vi "loadMapping.vi"(8 "error in (no error)":errorcluster, 9 "xmlPath":string, 10 "channel_configXML":refnum<class "NativeXML.lvclass">, 11 "Channel in":refnum<class "Channel.lvclass">) -> (0 "error out":errorcluster, 3 "Channel out":refnum<class "Channel.lvclass">)   [LabVIEW 2011, in "Tools.lvlib" / "DatabaseHelpers.lvlib" / "Channel.lvclass"]
uses:
  Channel.lvclass
  NativeXML/NativeXML.lvclass
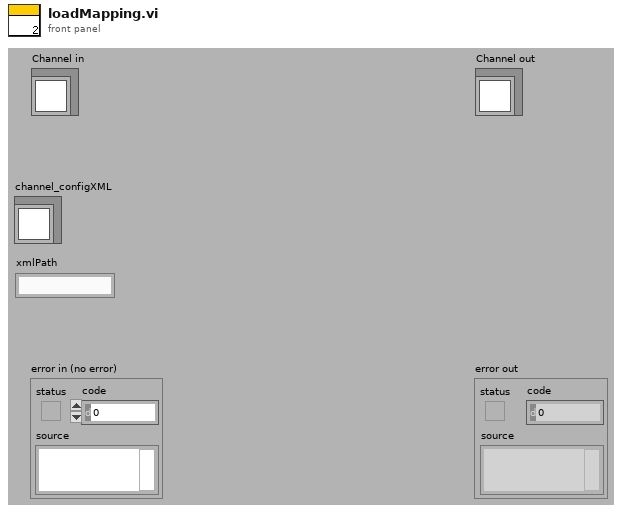
[diagram p1: front panel]
types:
  T1 = cluster{"Attribute String":string, "Value":string}
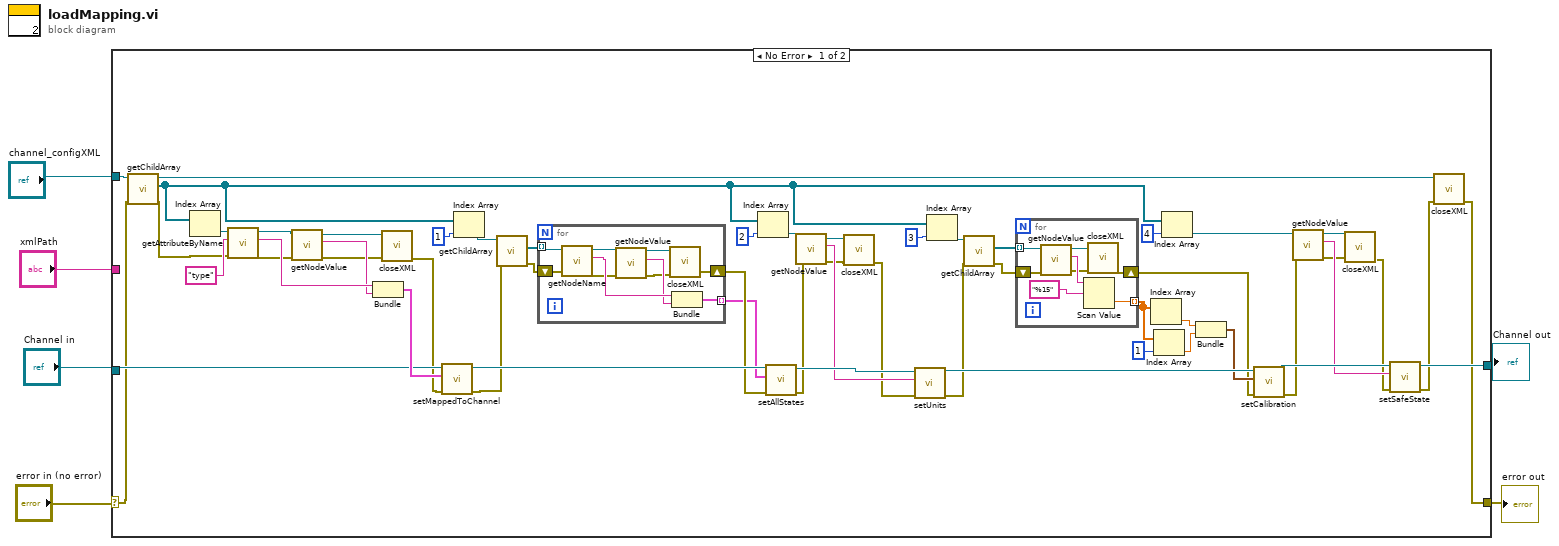
[diagram p0: block diagram]
diagram:
  n1 = case shown="No Error" "error in (no error)" {
    selector: "error in (no error)" -> [w41 w81]
    tunnel: [w7 w81] -> w4
    tunnel: "channel_configXML" -> [w43 _]
    tunnel: "Channel in" -> [w60 w80]
    tunnel: [w44 w80] -> w3
    tunnel: "xmlPath" -> [_ _]
    frame No Error {
      n2 = call "getChildArray.vi"("error in (no error)"=w41, "NativeXML in"=w43) -> ("error out"=w34:errorcluster, "childArray"=w42:refnum<class "NativeXML.lvclass">[], "NativeXML out"=w9:refnum<class "NativeXML.lvclass">)  [unwired: 7 in]
      n3 = Index Array(array=w42) -> (element=w39:refnum<class "NativeXML.lvclass">)  [unwired: 1 in]
      n4 = call "getAttributeByName.vi"("error in (no error)"=w34, "name"="type", "NativeXML in"=w39) -> ("error out"=w37:errorcluster, "Attribute String"=w38:string, "NativeXML out"=w36:refnum<class "NativeXML.lvclass">)  [unwired: 6 in]
      n5 = call "getNodeValue.vi"("error in (no error)"=w37, "NativeXML in"=w36) -> ("error out"=w17:errorcluster, "Value"=w35:string, "NativeXML out"=w18:refnum<class "NativeXML.lvclass">)  [unwired: 7 in]
      n6 = Bundle("Attribute String"=w38, "Value"=w35) -> (w61:T1)  [unwired: 1 in]
      n7 = call "closeXML.vi"("error in (no error)"=w17, "NativeXML in"=w18) -> ("error out"=w16:errorcluster)  [unwired: 9 in]
      n8 = call "setMappedToChannel.vi"("error in (no error)"=w16, "mappedTo"=w61, "Channel.lvclass in"=w60) -> ("error out"=w32:errorcluster, "Channel.lvclass out"=w58:refnum<class "Channel.lvclass">)  [unwired: 7 in]
      n9 = Index Array(array=w42, index=1) -> (element=w31:refnum<class "NativeXML.lvclass">)
      n10 = call "getChildArray.vi"("error in (no error)"=w32, "NativeXML in"=w31) -> ("error out"=w33:errorcluster, "childArray"=w30:refnum<class "NativeXML.lvclass">[])  [unwired: 7 in, 1 out]
      n11 = for {
        shift-right: [w70] -> w57
        shift-left: w33 -> [w78]
        tunnel: w30 -> [w77] mode=indexing
        tunnel: [w79] -> w45 mode=indexing
        n12 = call "getNodeName.vi"("error in (no error)"=w78, "NativeXML in"=w77) -> ("error out"=w74:errorcluster, "name"=w76:string, "NativeXML out"=w75:refnum<class "NativeXML.lvclass">)  [unwired: 7 in]
        n13 = call "getNodeValue.vi"("error in (no error)"=w74, "NativeXML in"=w75) -> ("error out"=w71:errorcluster, "Value"=w73:string, "NativeXML out"=w72:refnum<class "NativeXML.lvclass">)  [unwired: 7 in]
        n14 = call "closeXML.vi"("error in (no error)"=w71, "NativeXML in"=w72) -> ("error out"=w70:errorcluster)  [unwired: 9 in]
        n15 = Bundle("name"=w76, "Value"=w73) -> (w79:cluster{"name":string, "Value":string})  [unwired: 1 in]
      }
      n16 = Index Array(array=w42, index=2) -> (element=w29:refnum<class "NativeXML.lvclass">)
      n17 = call "setAllStates.vi"("error in (no error)"=w57, "states"=w45, "Channel.lvclass in"=w58) -> ("error out"=w28:errorcluster, "Channel.lvclass out"=w55:refnum<class "Channel.lvclass">)  [unwired: 7 in]
      n18 = call "getNodeValue.vi"("error in (no error)"=w28, "NativeXML in"=w29) -> ("error out"=w15:errorcluster, "Value"=w27:string, "NativeXML out"=w13:refnum<class "NativeXML.lvclass">)  [unwired: 7 in]
      n19 = call "closeXML.vi"("error in (no error)"=w15, "NativeXML in"=w13) -> ("error out"=w14:errorcluster)  [unwired: 9 in]
      n20 = call-dynamic "setUnits.vi"("error in (no error)"=w14, "units"=w27, "Channel.lvclass in"=w55) -> ("error out"=w25:errorcluster, "Channel.lvclass out"=w51:refnum<class "Channel.lvclass">)  [unwired: 7 in]
      n21 = Index Array(array=w42, index=3) -> (element=w24:refnum<class "NativeXML.lvclass">)
      n22 = call "getChildArray.vi"("error in (no error)"=w25, "NativeXML in"=w24) -> ("error out"=w26:errorcluster, "childArray"=w23:refnum<class "NativeXML.lvclass">[])  [unwired: 7 in, 1 out]
      n23 = for {
        tunnel: w23 -> [w67] mode=indexing
        tunnel: [w68] -> w53 mode=indexing
        shift-right: [w64] -> w19
        shift-left: w26 -> [w66]
        n24 = call "getNodeValue.vi"("error in (no error)"=w66, "NativeXML in"=w67) -> ("error out"=w63:errorcluster, "Value"=w65:string, "NativeXML out"=w62:refnum<class "NativeXML.lvclass">)  [unwired: 7 in]
        n25 = Scan Value(string=w65, format string="%15") -> (value=w68:dbl)  [unwired: 1 in, 1 out]
        n26 = call "closeXML.vi"("error in (no error)"=w63, "NativeXML in"=w62) -> ("error out"=w64:errorcluster)  [unwired: 9 in]
      }
      n27 = Index Array(array=w53) -> (element=w50:dbl)  [unwired: 1 in]
      n28 = Index Array(array=w53, index=1) -> (element=w49:dbl)
      n29 = Index Array(array=w42, index=4) -> (element=w22:refnum<class "NativeXML.lvclass">)
      n30 = Bundle(w50, w49) -> (w48:cluster{dbl, dbl})  [unwired: 1 in]
      n31 = call "setCalibration.vi"("error in (no error)"=w19, "calibration"=w48, "Channel.lvclass in"=w51) -> ("error out"=w21:errorcluster, "Channel.lvclass out"=w46:refnum<class "Channel.lvclass">)  [unwired: 7 in]
      n32 = call "getNodeValue.vi"("error in (no error)"=w21, "NativeXML in"=w22) -> ("error out"=w11:errorcluster, "Value"=w20:string, "NativeXML out"=w12:refnum<class "NativeXML.lvclass">)  [unwired: 7 in]
      n33 = call "closeXML.vi"("error in (no error)"=w11, "NativeXML in"=w12) -> ("error out"=w10:errorcluster)  [unwired: 9 in]
      n34 = call "setSafeState.vi"("error in (no error)"=w10, "safe_state"=w20, "Channel.lvclass in"=w46) -> ("error out"=w8:errorcluster, "Channel.lvclass out"=w44:refnum<class "Channel.lvclass">)  [unwired: 7 in]
      n35 = call "closeXML.vi"("error in (no error)"=w8, "NativeXML in"=w9) -> ("error out"=w7:errorcluster)  [unwired: 9 in]
    }
    frame Error {
    }
  }
  "error out" <- w4
  "Channel out" <- w3
